vi "ProcessName.vi"() -> (1 "process name":string)   [LabVIEW 2017, in "CmsFpgaBitfileManager.lvlib"]
uses:
  <vilib>/addons/InsightCM/Devices/Shared/Cms/CmsFpgaBitfileManager/CmsFpgaBitfileManager.lvlib
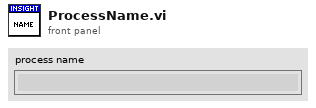
[diagram p1: front panel]
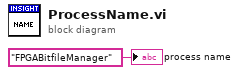
[diagram p0: block diagram]
diagram:
  "process name" <- "FPGABitfileManager" ("ProcessName")
